vi "Test RC.vi"(8 "error in (no error)":errorcluster, 11 "RC Type":T1=enum."ZMQ") -> (0 "error out":errorcluster)   [LabVIEW 2019]
uses:
  <userlib>/LevyLab/RemoteControl/RemoteControl/Typedefs/RC Com Type--enum.ctl
  <userlib>/LevyLab/RemoteControl/RemoteControl.ZMQ/RemoteControl.ZMQ.lvclass
  C:/Program Files (x86)/National Instruments/LabVIEW 2019/user.lib/LevyLab/RemoteControl/RemoteControl/RemoteControl.lvclass
  <userlib>/LevyLab/RemoteControl.STM/RemoteControl.STM.lvclass
  <vilib>/addons/_JKI Toolkits/Caraya/classes/Assert/Assert Not Error.vi
  <userlib>/LevyLab/RemoteControl/RemoteControl/RemoteControl.lvclass
  <vilib>/addons/_JKI Toolkits/Caraya/classes/Assert/Assert.lvclass
  <vilib>/addons/_JKI Toolkits/Caraya/classes/Test/Test.lvclass
  C:/Program Files (x86)/National Instruments/LabVIEW 2019/vi.lib/JKI/JKI SMO/SMO/SMO.lvclass
panel:
  # "1. Choose RC Type\n2. Run This VI\n3. An orange server will open. Three pink clients will then open. Watch the messasges.\n4. When you are satisfied:\n- first stop the clients and\n- then stop the server."
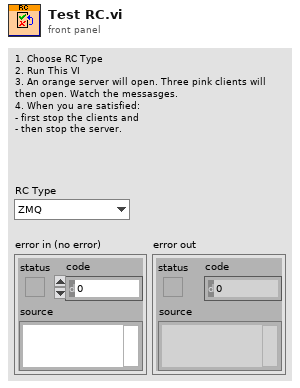
[diagram p1: front panel]
types:
  T1 = typedef "RemoteControl.lvclass/RC Com Type--enum.ctl" = enum16{"RC", "STM", "ZMQ"}
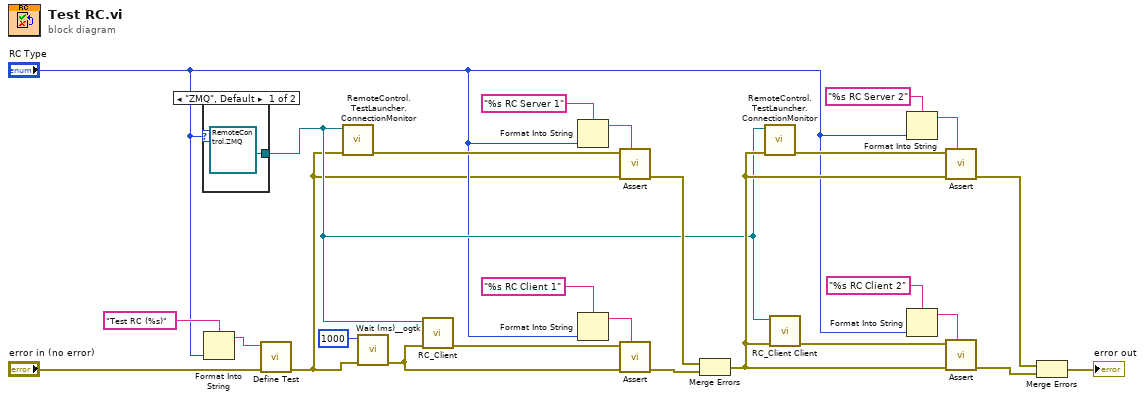
[diagram p0: block diagram]
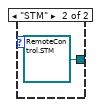
[diagram p2: hidden frame]
diagram:
  n1 = case shown="\"ZMQ\", Default" "RC Type" {
    tunnel: [refnum<class "RemoteControl.ZMQ.lvclass"> refnum ("RemoteControl.ZMQ.lvclass") refnum<class "RemoteControl.STM.lvclass"> refnum ("RemoteControl.STM.lvclass")] -> w5
    frame "ZMQ", Default {
    }
    frame "STM" {
    }
  }
  n2 = Format Into String(format string="Test RC (%s)", "RC Type") -> (resulting string=w24:string)  [unwired: 2 in, 1 out]
  n3 = call <vilib>:"Define Test.vi"("error in (no error)"="error in (no error)", "Label (VI Title)"=w24) -> ("error out"=w3:errorcluster)  [unwired: 8 in, 1 out]
  n4 = call <userlib>:"RemoteControl.TestLauncher.ConnectionMonitor.vi"("error in (no error)"=w3, "RemoteControl in"=w5) -> ("error out"=w22:errorcluster)  [unwired: 9 in]
  n5 = call <userlib>:"Wait (ms)__ogtk.vi"("error in (no error)"=w3, "milliseconds to wait"=u32 1000) -> ("error out"=w2:errorcluster)  [unwired: 8 in, 1 out]
  n6 = call <userlib>:"RC_Client.vi"("error in (no error)"=w2, "RemoteControl in"=w5) -> ("error out"=w21:errorcluster)  [unwired: 9 in]
  n7 = Format Into String(format string="%s RC Server 1", "RC Type") -> (resulting string=w14:string)  [unwired: 2 in, 1 out]
  n8 = Format Into String(format string="%s RC Client 1", "RC Type") -> (resulting string=w10:string)  [unwired: 2 in, 1 out]
  n9 = call-poly <vilib>:"Assert.vi"("Label"=w14, "error in (no error)"=w3, "Not Error?"=w22) -> ("error out"=w18:errorcluster)  [unwired: 7 in, 1 out]
  n10 = call-poly <vilib>:"Assert.vi"("Label"=w10, "error in (no error)"=w2, "Not Error?"=w21) -> ("error out"=w17:errorcluster)  [unwired: 7 in, 1 out]
  n11 = Merge Errors(w18, w17) -> (w6:errorcluster)
  n12 = call <userlib>:"RemoteControl.TestLauncher.ConnectionMonitor.vi"("error in (no error)"=w6, "RemoteControl in"=w5) -> ("error out"=w19:errorcluster)  [unwired: 9 in]
  n13 = call <userlib>:"RC_Client Client.vi"("error in (no error)"=w6, "RemoteControl in"=w5) -> ("error out"=w20:errorcluster)  [unwired: 9 in]
  n14 = Format Into String(format string="%s RC Server 2", "RC Type") -> (resulting string=w12:string)  [unwired: 2 in, 1 out]
  n15 = Format Into String(format string="%s RC Client 2", "RC Type") -> (resulting string=w8:string)  [unwired: 2 in, 1 out]
  n16 = call-poly <vilib>:"Assert.vi"("Label"=w12, "error in (no error)"=w6, "Not Error?"=w19) -> ("error out"=w16:errorcluster)  [unwired: 7 in, 1 out]
  n17 = call-poly <vilib>:"Assert.vi"("Label"=w8, "error in (no error)"=w6, "Not Error?"=w20) -> ("error out"=w7:errorcluster)  [unwired: 7 in, 1 out]
  n18 = Merge Errors(w16, w7) -> (→"error out":errorcluster)
